vi "ZeroifTrue.vi"(1 "Input":dbl) -> (0 "Output":dbl)   [LabVIEW 2015]
uses:
  <vilib>/Rock Robotics/WPI/Solenoid/Deprecated/WPI_SolenoidGetBool.vi
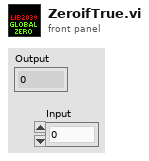
[diagram p1: front panel]
types:
  T1 = typedef "WPI_SolenoidDevRef.ctl" = cluster{"DevStatus":errorcluster, "Pneumatics Control Module":u8, "Forward Solenoid Channel":T2, "Reverse Solenoid Channel":T2}
  T2 = typedef "WPI_SolenoidChannel.ctl" = enum8{"Solenoid 0", "Solenoid 1", "Solenoid 2", "Solenoid 3", "Solenoid 4", "Solenoid 5", "Solenoid 6", "Solenoid 7", "Invalid"}
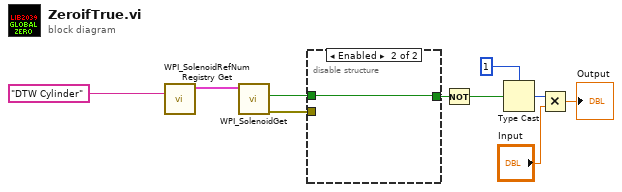
[diagram p0: block diagram]
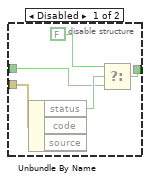
[diagram p2: hidden frame]
diagram:
  n1 = call <vilib>:"WPI_SolenoidRefNum Registry Get.vi"("refnum name"="DTW Cylinder") -> ("SolenoidDevRef"=w5:T1)  [unwired: 9 in, 1 out]
  n2 = call-poly <vilib>:"WPI_SolenoidGet.vi"("SolenoidDevRef"=w5) -> ("error out"=w3:errorcluster, "Value"=w2:bool)  [unwired: 8 in, 1 out]
  n3 = disable-structure shown="Enabled" {
    disable-tunnel: w3 -> [w15 _]
    disable-tunnel: w2 -> [w12 w16]
    disable-tunnel: [w11 w16] -> w1
    frame Disabled {
      n4 = Unbundle By Name(w15) -> ("status"=w14:bool)  [unwired: 2 out]
      n5 = Select(t=FALSE, s=w14, f=w12) -> (s? t:f=w11:bool)
    }
    frame Enabled {
    }
  }
  n6 = Not(x=w1) -> (.not. x?=w9:bool)
  n7 = Type Cast(type=1, x=w9) -> (*(type *) &x=w8:i32)
  n8 = Multiply(x=w8, y="Input") -> (x*y=→"Output":dbl)
